vi "Write String.vi"(8 "error in (no error)":errorcluster, 10 "String":string, 11 "String STEP in":refnum<class "String STEP.lvclass">) -> (0 "error out":errorcluster, 3 "String STEP out":refnum<class "String STEP.lvclass">)   [LabVIEW 2014, in "String STEP.lvclass"]
uses:
  String STEP.lvclass
  String STEP.lvclass/String STEP.ctl
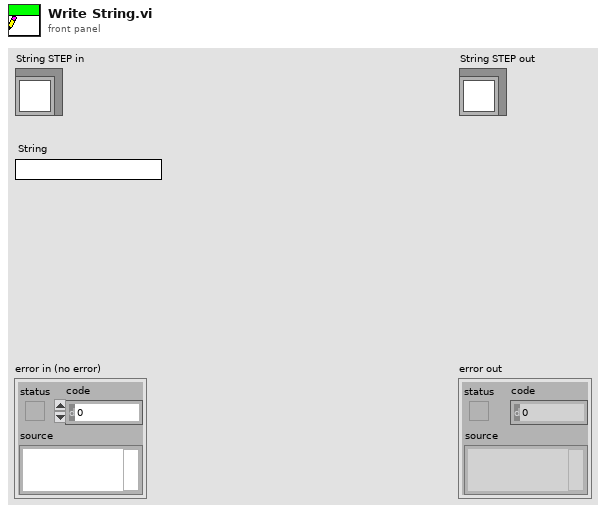
[diagram p1: front panel]
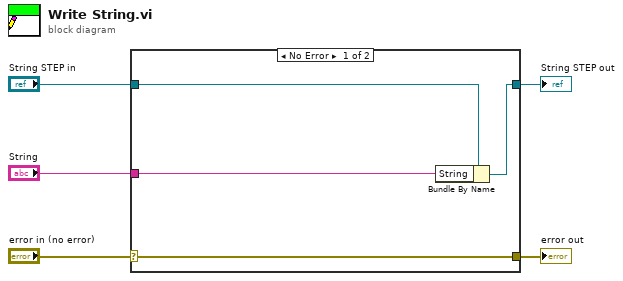
[diagram p0: block diagram]
diagram:
  n1 = case shown="No Error" "error in (no error)" {
    selector: "error in (no error)" -> [w9 w10]
    tunnel: [w9 w10] -> w4
    tunnel: [w7 w11] -> w2
    tunnel: "String STEP in" -> [w8 w11]
    tunnel: "String" -> [w6 _]
    frame No Error {
      n2 = Bundle By Name(cluster=w8, "String"=w6) -> (w7:refnum<class "String STEP.lvclass">)
    }
    frame Error {
    }
  }
  "error out" <- w4
  "String STEP out" <- w2
